vi "UNIT.vi"(8 "Error in (no error)":errorcluster, 9 "Units":string="T", 10 "Function":T1(ring)=enum."Units query", 11 "VISA resource":refnum<visa-resource-name>) -> (0 "Error out":errorcluster, 2 "Units out":string, 3 "Dup VISA resource":refnum<visa-resource-name>)   [LabVIEW 2010]
doc: "Copyright (c) 2012 Metrolab Technology SA, Plan-les-Ouates, Geneva, Switzerland\nSets the units in which measurements are returned, or queries the currently selected units.\nNote that units are only used if FORMat is Ascii and CALibration:STATe is On."
panel:
  # "UNIT"
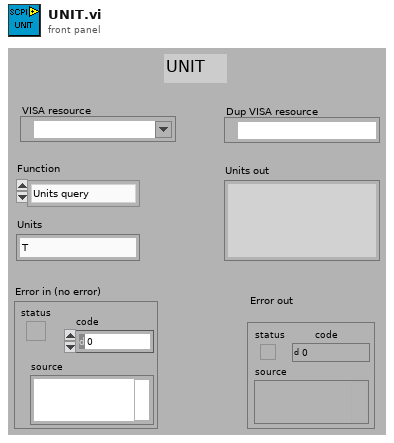
[diagram p1: front panel]
types:
  T1 = enum16{"Set units", "Units query", "Units all query"}
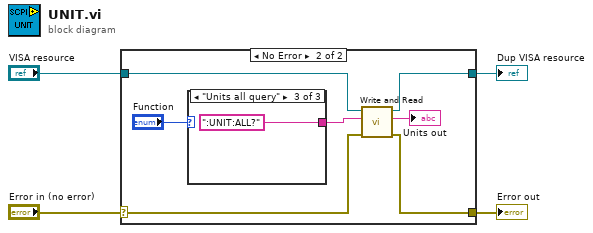
[diagram p0: block diagram]
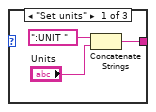
[diagram p3: hidden frame]
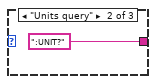
[diagram p4: hidden frame]
diagram:
  n1 = case shown="No Error" "Error in (no error)" {
    selector: "Error in (no error)" -> [w5 w10]
    tunnel: "VISA resource" -> [w6 w13]
    tunnel: [w6 w9] -> w1
    tunnel: [w5 w8] -> w4
    frame Error {
    }
    frame No Error {
      n2 = case shown="\"Units all query\"" "Function" {
        tunnel: [w16 ":UNIT?" ":UNIT:ALL?"] -> w7
        frame "Set units" {
          n3 = Concatenate Strings(":UNIT " ("string"), "Units") -> (w16:string)
        }
        frame "Units query" {
        }
        frame "Units all query" {
        }
      }
      n4 = call "Write and Read.vi"("Error in (no error)"=w10, "Command"=w7, "VISA resource"=w13) -> ("Error out"=w8:errorcluster, "Response"=→"Units out":string, "Dup VISA resource"=w9:refnum<visa-resource-name>)  [unwired: 4 in, 2 out]
    }
  }
  "Error out" <- w4
  "Dup VISA resource" <- w1
